vi "Configure Mixer Level Offset.vi"(8 "error in (no error)":errorcluster, 9 "Mixer Level Offset (8.0)":dbl=8.0 format="%^.3e", 10 "Instance (1)":T1=1, 11 "VISA resource name":refnum<visa-resource-name>) -> (0 "error out":errorcluster, 3 "VISA resource name out":refnum<visa-resource-name>)   [LabVIEW 2015, in "Rohde&Schwarz CMXP NR FR2 Measurement.lvlib"]
doc: "Varies the input level of the mixer in the analyzer path.\n\nAttribute:\nRSCMXPNRFR2M_ATTR_MIXER_LEVEL_OFFSET\n\nRemote-control command:\nCONFigure:NRMMw:MEAS<i>:RFSettings:MLOFfset"
uses:
  <instrlib>/Rohde&Schwarz CMXP NR FR2 Measurement/Rohde&Schwarz CMXP NR FR2 Measurement.lvlib
  <instrlib>/Rohde&Schwarz CMXP NR FR2 Measurement/Private/_Instance.ctl
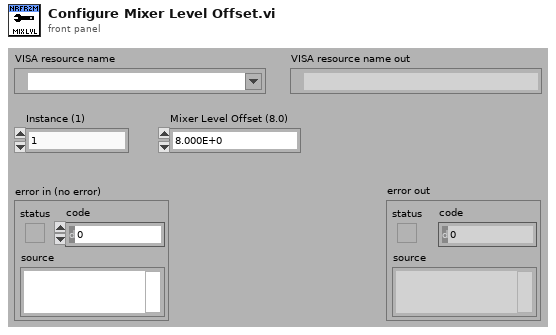
[diagram p1: front panel]
types:
  T1 = typedef "Rohde&Schwarz CMXP NR FR2 Measurement.lvlib/_Instance.ctl" = i32
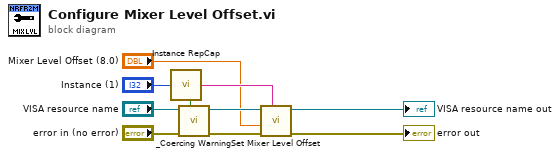
[diagram p0: block diagram]
diagram:
  n1 = call <instrlib>:"Instance RepCap.vi"("Instance In"="Instance (1)") -> ("In Range?"=w6:bool, "RepCap Identifier Out"=w5:string)  [unwired: 1 in]
  n2 = call <instrlib>:"_Coercing Warning.vi"("In Range?"=w6, "error in (no error)"="error in (no error)", "VISA resource name"="VISA resource name") -> ("error out"=w4:errorcluster, "VISA resource name out"=w3:refnum<visa-resource-name>)  [unwired: 7 in]
  n3 = call "Set Mixer Level Offset"("Repeated Capabilities"=w5, "error in (no error)"=w4, "Mixer Level Offset (0.0)"="Mixer Level Offset (8.0)", "instrument handle"=w3) -> ("error out"=→"error out":errorcluster, "instrument handle out"=→"VISA resource name out":refnum<visa-resource-name>)  [unwired: 6 in]
